vi "Manipulator Controller.vi"(8 "error in":errorcluster) -> ()   [LabVIEW 2018]
doc: "This VI executes continuously carrying out the current operation and responding to updates or new operations. It will often contain the timing or control code that is difficult to place directly in TeleOp. This VI generally opens all sensors and motors and isolates the rest of the robot code from knowing how the operations are carried out."
uses:
  <vilib>/Rock Robotics/WPI/Framework/Completion Status.ctl
  Manipulator Setpoints.ctl
  Manipulator Operations.ctl
  <vilib>/Rock Robotics/WPI/SafetyOutput/WPI_SafetyOutputConfigMenu.ctl
  <vilib>/addons/control/pid/NI_PID_pid.lvlib
  <vilib>/addons/control/pid/pid.llb/PID (DBL).vi
panel:
  in  "upper angle":dbl=0.35
  in  "lower angle":dbl=0.2
  in  "\"power\" for the hatch motor":dbl=0.75
  in  "margin of error":dbl=0.1
  in  "PID gains":T1={"proportional gain (Kc)"=1.0, "integral time (Ti, min)"=0.01, "derivative time (Td, min)"=0.0} {"derivative time (Td, min)" format="%.3f"; "integral time (Ti, min)" format="%.3f"; "proportional gain (Kc)" format="%.3f"}
  in  "Interactive Values":T2
  out "Current\nCmd":string
  in  "Buttons":cluster{"Execute Cmd":bool, "Abort Cmd":bool}
  out "Command Timing":cluster{"Start Time (ms)":u32, "Iterations":i32}
  out "Status":T4
  # "Tip: It may be helpful to observe inputs and sensor values.\nYou may also want to display tuning or debugging controls."
  # "Interactive Command: You may fill in the settings for a command\nand schedule it with the Execute button. You can observe and abort\nany command while fine tuning the code for the controller."
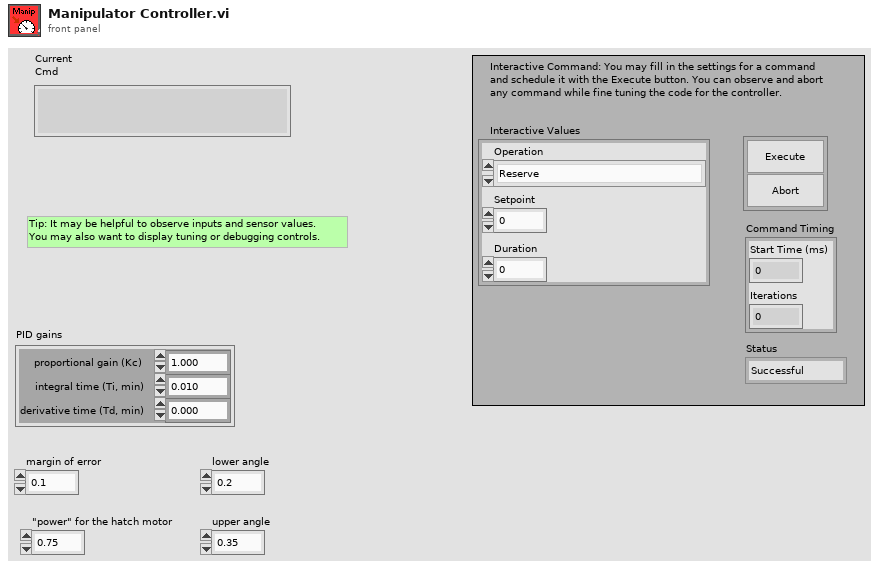
[diagram p1: front panel]
types:
  T1 = cluster{"proportional gain (Kc)":dbl, "integral time (Ti, min)":dbl, "derivative time (Td, min)":dbl}
  T2 = typedef "Manipulator Setpoints.ctl" = cluster{"Operation":T3, "Setpoint":dbl, "Duration":dbl}
  T3 = typedef "Manipulator Operations.ctl" = enum16{"Reserve", "Read Current", "Immediate", "LowerArm", "RaiseArm", "HoldingCover"}
  T4 = typedef "Completion Status.ctl" = enum16{"Successful", "Aborted", "Incomplete"}
  T5 = typedef "WPI_SafetyOutputConfigMenu.ctl" = enum16{"Enable", "Disable"}
  T6 = typedef "WPI_MotorControlDeviceRef.ctl" = cluster{"DeviceStatus":errorcluster, "Type":T7, "PWM":cluster{"PWM Channel":T8, "DeadBand":T9}, "CAN":cluster{"Device Number":u8, "SetOutput VI Ref":variant, "GetOutput VI Ref":variant, "Enable VI Ref":variant, "Disable VI Ref":variant, "Data":variant}, "Invert":bool, "DIO PWM":cluster{"PWM \"Enable\" Channel":T8, "DIOChannel":T10, "PWM Rate":dbl}}
  T7 = typedef "WPI_MotorControlType.ctl" = enum16{"PWM", "CAN", "DIO PWM"}
  T8 = typedef "FPGA_DIOPWMChannel.ctl" = enum8{"PWM 0", "PWM 1", "PWM 2", "PWM 3", "PWM 4", "PWM 5", "PWM 6", "PWM 7", "PWM 8", "PWM 9", "PWM MXP 0", "PWM MXP 1", "PWM MXP 2", "PWM MXP 3", "PWM MXP 4", "PWM MXP 5", "PWM MXP 6", "PWM MXP 7", "PWM MXP 8", "PWM MXP 9", "Invalid"}
  T9 = typedef "WPI_PWMDeadband.ctl" = cluster{"Name":string, "maxPositivePwm":i32, "minPositivePwm":i32, "centerPwm":i32, "maxNegativePwm":i32, "minNegativePwm":i32, "angularRange":u16}
  T10 = typedef "FPGA_DIOChannel.ctl" = enum8{"DIO 0", "DIO 1", "DIO 2", "DIO 3", "DIO 4", "DIO 5", "DIO 6", "DIO 7", "DIO 8", "DIO 9", "DIO MXP 0", "DIO MXP 1", "DIO MXP 2", "DIO MXP 3", "DIO MXP 4", "DIO MXP 5", "DIO MXP 6", "DIO MXP 7", "DIO MXP 8", "DIO MXP 9", "DIO MXP 10", "DIO MXP 11", "DIO MXP 12", "DIO MXP 13", "DIO MXP 14", "DIO MXP 15", "SPI Port CS1", "SPI Port CS2", "SPI Port CS3", "SPI Port MISO", "SPI Port MOSI", "Invalid"}
  T11 = typedef "Command Status Info.ctl" = cluster{"Name":string, "Status":T4, "notifier out":T12}
  T12 = typedef "Completion Notifier.ctl" = refnum<notifier>
  T13 = cluster{"Current Command":T2, "Command Timing":cluster{"Start Time (ms)":u32, "Iterations":i32}, "Command Arguments":cluster{"Command Info":T11, "Description":string, "Default Command":T2, "queue out":refnum<queue>, "Subsystem Name":string}}
  T14 = typedef "WPI_PotentiometerDevRef.ctl" = cluster{"DevStatus":errorcluster, "Analog Channel":T15, "Invert Output":bool}
  T15 = typedef "FPGA_AIChannel.ctl" = enum8{"AI 0", "AI 1", "AI 2", "AI 3", "AI MXP 0", "AI MXP 1", "AI MXP 2", "AI MXP 3", "Invalid"}
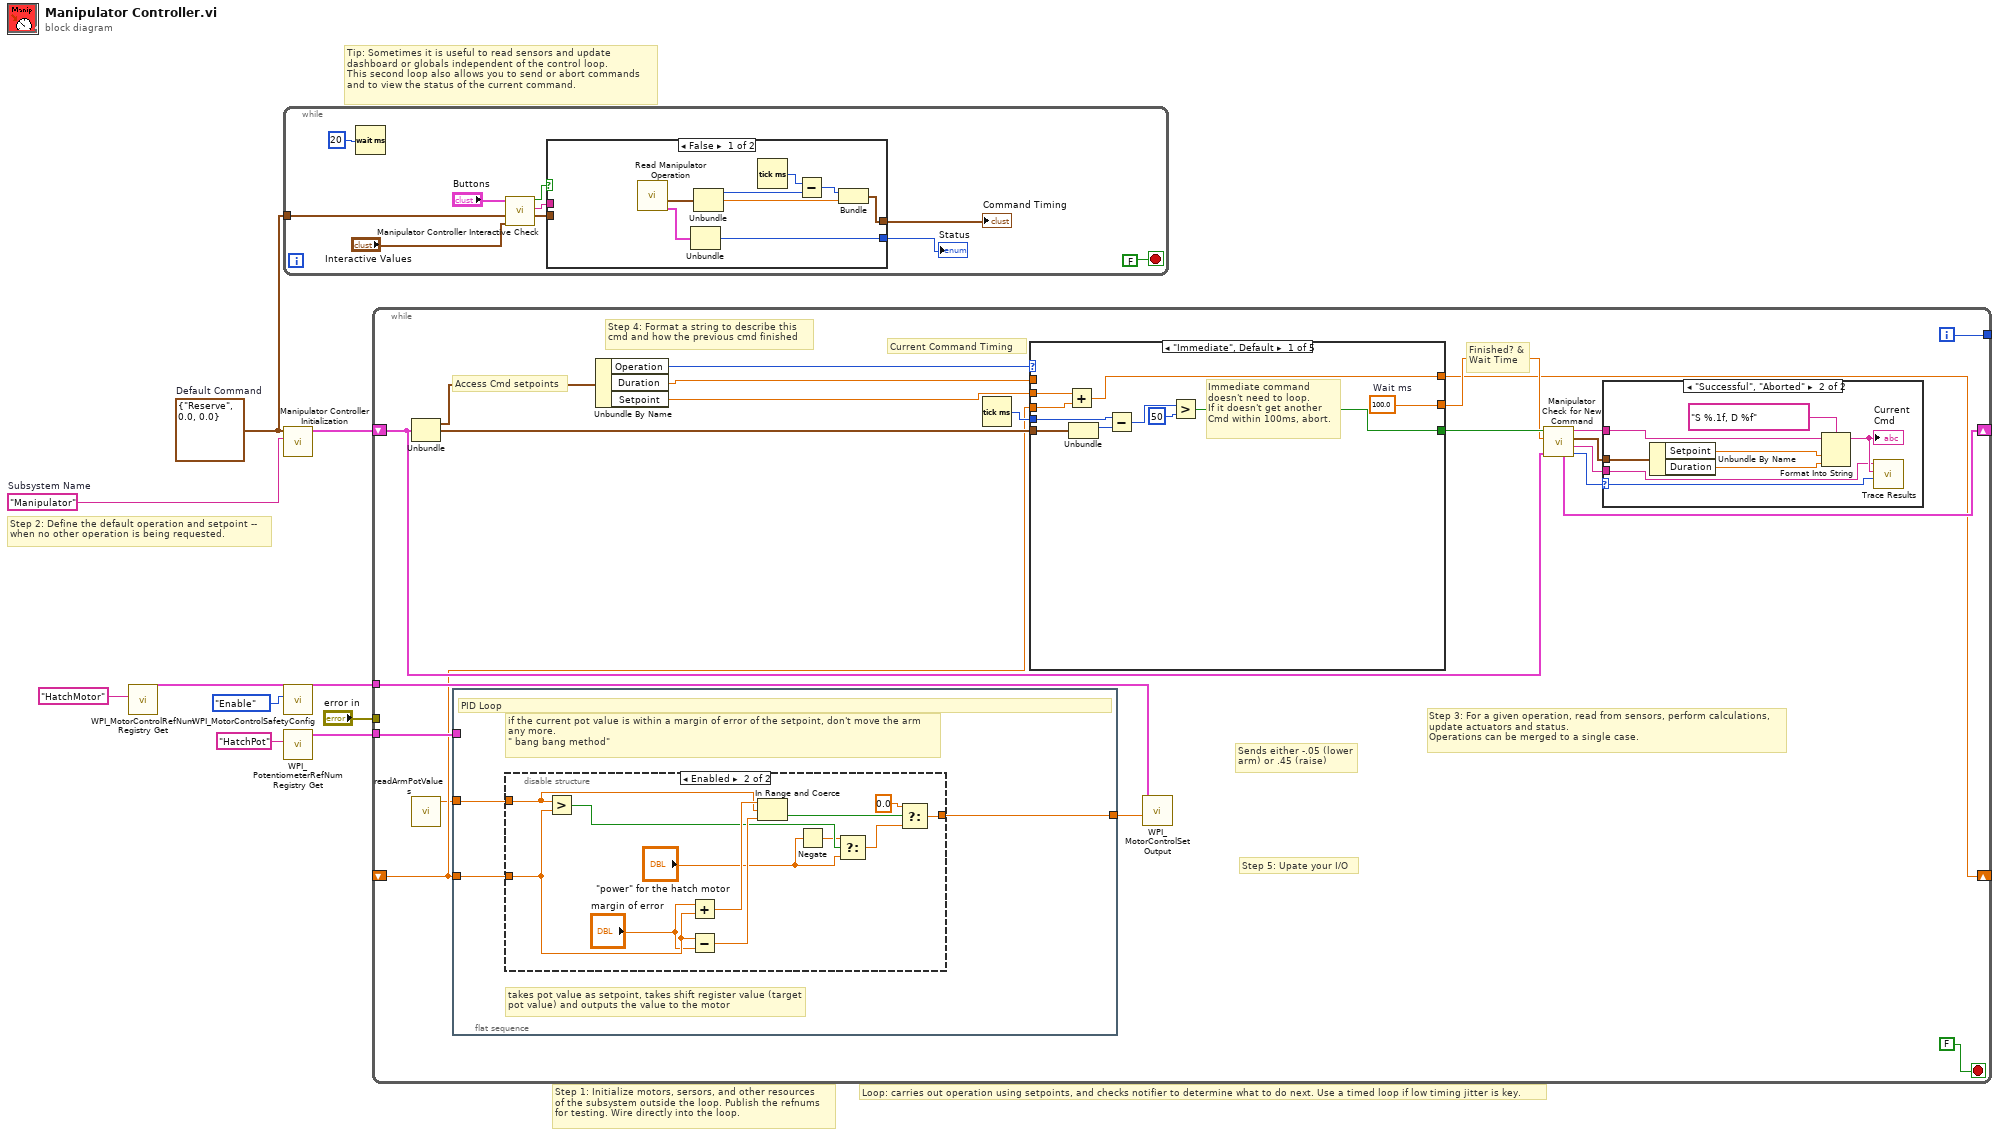
[diagram p0: block diagram]
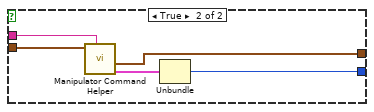
[diagram p2: hidden frame]
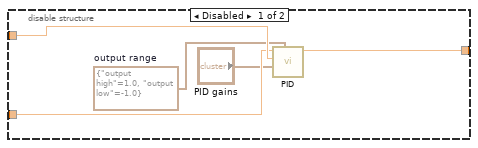
[diagram p3: hidden frame]
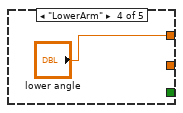
[diagram p7: hidden frame]
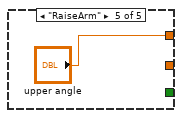
[diagram p8: hidden frame]
diagram:
  w7 = T2 {"Operation"=enum."Reserve", "Setpoint"=0.0, "Duration"=0.0}  # Default Command
  w8 = "Manipulator"  # Subsystem Name
  # "Tip: Sometimes it is useful to read sensors and update\ndashboard or globals independent of the control loop.\nThis second loop also allows you to send or abort commands\nand to view the status of the current command."
  # "Step 2: Define the default operation and setpoint --\nwhen no other operation is being requested."
  # "Step 1: Initialize motors, sersors, and other resources\nof the subsystem outside the loop. Publish the refnums\nfor testing. Wire directly into the loop."
  # "Loop: carries out operation using setpoints, and checks notifier to determine what to do next. Use a timed loop if low timing jitter is key."
  n1 = call <vilib>:"WPI_MotorControlRefNum Registry Get.vi"("refnum name"="HatchMotor") -> ("MotorControlDevRef"=w6:T6)  [unwired: 9 in, 1 out]
  n2 = while {
    tunnel: w7 -> [w17]
    stop <- FALSE stop-if-true
    n3 = Wait (ms)(milliseconds to wait=u32 20) -> ()  [unwired: 1 out]
    n4 = call "Manipulator Controller Interactive Check.vi"("Interactive Command in"="Interactive Values", "Default Command"=w17, "Buttons"="Buttons") -> ("Interactive Command out"=w14:T2, "Trace String"=w15:string, "Schedule"=w16:bool)  [unwired: 6 in]
    n5 = case shown="False" w16 {
      tunnel: [w28 w33] -> w13
      tunnel: w14 -> [_ w31]
      tunnel: [w24 w29] -> w12
      tunnel: w15 -> [_ w32]
      frame False {
        n6 = call "Read Manipulator Operation.vi"() -> ("Command Info"=w21:T11, "SubSystem Data"=w22:T2)  [unwired: 9 in, 1 out]
        n7 = Unbundle(w21) -> ("Status"=w28:T4)  [unwired: 2 out]
        n8 = Unbundle(w22) -> ("Operation"=w27:T3, "Setpoint"=w25:dbl)  [unwired: 1 out]
        n9 = Tick Count (ms)() -> (millisecond timer value=w23:u32)
        n10 = Subtract(x=w23, y=w27) -> (x-y=w26:u32)
        n11 = Bundle(w26, "Setpoint"=w25) -> (w24:cluster{u32, "Setpoint":dbl})  [unwired: 1 in]
      }
      frame True {
        n12 = call "Manipulator Command Helper.vi"("Description"=w32, "SubSystem Data"=w31) -> ("Command Info Out"=w30:T11, "Command Timing"=w29:cluster{"Start Time (ms)":u32, "Iterations":i32})  [unwired: 7 in, 1 out]
        n13 = Unbundle(w30) -> ("Status"=w33:T4)  [unwired: 2 out]
      }
    }
    "Status" <- w13
    "Command Timing" <- w12
  }
  n14 = call "Manipulator Controller Initialization.vi"("Subsystem Name"=w8, "Default Command"=w7) -> ("Current Command"=w9:T13)  [unwired: 9 in]
  n15 = call <vilib>:"WPI_MotorControlSafetyConfig.vi"("mode"=WPI_SafetyOutputConfigMenu."Enable", "MotorControlDevRef"=w6) -> ("MotorControlDevRef"=w4:T6)  [unwired: 8 in, 1 out]
  n16 = call <vilib>:"WPI_PotentiometerRefNum Registry Get.vi"("refnum name"="HatchPot") -> ("PotDevRef"=w2:T14)  [unwired: 9 in, 1 out]
  n17 = while {
    shift-right: [w47] -> _
    shift-left: w9 -> [w40]
    tunnel: [w54] -> _
    tunnel: "error in" -> [_]
    tunnel: w4 -> [w36]
    shift-right: [w39] -> _
    shift-left: _ -> [w35]
    tunnel: w2 -> [w38]
    i -> [w54]
    stop <- FALSE stop-if-true
    # "Sends either -.05 (lower\narm) or .45 (raise)"
    # "Step 5: Upate your I/O"
    # "Step 4: Format a string to describe this\ncmd and how the previous cmd finished"
    # "Current Command Timing"
    # "Access Cmd setpoints"
    # "Finished? &\nWait Time"
    # "Step 3: For a given operation, read from sensors, perform calculations,\nupdate actuators and status.\nOperations can be merged to a single case."
    n18 = Unbundle(w40) -> ("Current Command"=w53:T2, "Command Timing"=w49:cluster{"Start Time (ms)":u32, "Iterations":i32})  [unwired: 1 out]
    n19 = call "readArmPotValues.vi"() -> ("Normalized Value"=w34:dbl)  [unwired: 11 in]
    n20 = flat-sequence {
      tunnel: w35 -> [w57]
      tunnel: w38 -> [_]
      tunnel: w34 -> [w58]
      tunnel: [w56] -> w37
      frame #0 {
        # "if the current pot value is within a margin of error of the setpoint, don't move the arm\nany more.\n\" bang bang method\""
        # "takes pot value as setpoint, takes shift register value (target\npot value) and outputs the value to the motor"
        # "PID Loop"
        n21 = disable-structure shown="Enabled" {
          disable-tunnel: w58 -> [w63 w68]
          disable-tunnel: w57 -> [w62 w67]
          disable-tunnel: [w59 w69] -> w56
          frame Disabled {
            w60 = cluster{"output high":dbl, "output low":dbl} {"output high"=1.0, "output low"=-1.0}  # output range
            n22 = call-poly <vilib>:"PID.vi"("output range"=w60, "PID gains"="PID gains", "process variable"=w63, "setpoint"=w62) -> ("output"=w59:dbl)  [unwired: 6 in, 1 out]
          }
          frame Enabled {
            n23 = Greater?(x=w68, y=w67) -> (0:w71:bool)
            n24 = Add(x="margin of error", y=w67) -> (x+y=w75:dbl)
            n25 = Subtract(x=w67, y="margin of error") -> (x-y=w74:dbl)
            n26 = In Range and Coerce(upper limit=w75, x=w68, lower limit=w74) -> (In Range?=w73:bool)  [unwired: 1 out]
            n27 = Negate(x="\"power\" for the hatch motor") -> (-x=w64:dbl)
            n28 = Select(t=w64, s=w71, f="\"power\" for the hatch motor") -> (s? t:f=w70:dbl)
            n29 = Select(t=0.0, s=w73, f=w70) -> (s? t:f=w69:dbl)
          }
        }
      }
    }
    n30 = Unbundle By Name(w53) -> ("Operation"=w52:T3, "Duration"=w51:dbl, "Setpoint"=w48:dbl)
    n31 = Tick Count (ms)() -> (millisecond timer value=w50:u32)
    n32 = case shown="\"Immediate\", Default" w52 {
      tunnel: [w93 _ _ _ _] -> w45
      tunnel: [w87 _ _ _ _] -> w46
      tunnel: w49 -> [w89 _ _ _ _]
      tunnel: w51 -> [_ _ _ _ _]
      tunnel: w50 -> [w88 _ _ _ _]
      tunnel: w48 -> [w86 _ _ _ _]
      tunnel: [w84 w94 w95 "lower angle" "upper angle"] -> w39
      tunnel: w35 -> [w85 w94 w95 _ _]
      frame "Immediate", Default {
        w93 = 100.0  # Wait ms
        # "Immediate command\ndoesn't need to loop.\nIf it doesn't get another\nCmd within 100ms, abort."
        n33 = Add(x=w86, y=w85) -> (x+y=w84:dbl)
        n34 = Unbundle(w89) -> ("Start Time (ms)"=w92:u32)  [unwired: 1 out]
        n35 = Subtract(x=w88, y=w92) -> (x-y=w91:u32)
        n36 = Greater?(x=w91, y=u8 50 ("Left Motor")) -> (0:w87:bool)
      }
      frame "Reserve" {
        # "If loop needs to poll sensors or other\nvalues, use a timeout value. -1 waits for\nnext command to be sent."
      }
      frame "Read Current" {
      }
      frame "LowerArm" {
      }
      frame "RaiseArm" {
      }
    }
    n37 = call <vilib>:"WPI_MotorControlSetOutput.vi"("Output"=w37, "MotorControlDevRef"=w36) -> ()  [unwired: 7 in, 3 out]
    n38 = call "Manipulator Check for New Command.vi"("Current Command"=w40, "Wait time (ms)"=w45, "Finished?"=w46) -> ("Completion"=w41:T4, "Subsystem Name"=w42:string, "Current Command"=w43:T2, "Initial Trace String"=w44:string, "NextCommand"=w47:T13)  [unwired: 4 in]
    n39 = case shown="\"Successful\", \"Aborted\"" w41 {
      selector: w41 -> [_ w83]
      tunnel: w44 -> [_ w79]
      tunnel: w43 -> [_ w80]
      tunnel: w42 -> [_ w76]
      frame "Incomplete", Default {
        # "Continuing current command"
      }
      frame "Successful", "Aborted" {
        # "Report and setup for next command"
        n40 = Unbundle By Name(w80) -> ("Setpoint"=w82:dbl, "Duration"=w77:dbl)
        n41 = Format Into String(format string="S %.1f, D %f", initial string=w79, w82, w77) -> (resulting string=w78:string)  [unwired: 1 in, 1 out]
        "Current\nCmd" <- w78
        n42 = call <vilib>:"Trace Results.vi"("Status of previous command"=w83, "Description"=w78, "Subsystem"=w76) -> ()  [unwired: 9 in]
      }
    }
  }
